vi "binning.vi"(10 "Number to bin":i32=2, 11 "path":path) -> ()   [LabVIEW 2023]
uses:
  <vilib>/Utility/file.llb/Read Delimited Spreadsheet (I64).vi
  <vilib>/Utility/file.llb/Write Delimited Spreadsheet (I64).vi
panel:
  out "Horizontal Fill Slide":dbl(slide) scale=0.0..100.0
  out "error out":errorcluster
  in  "error in":errorcluster
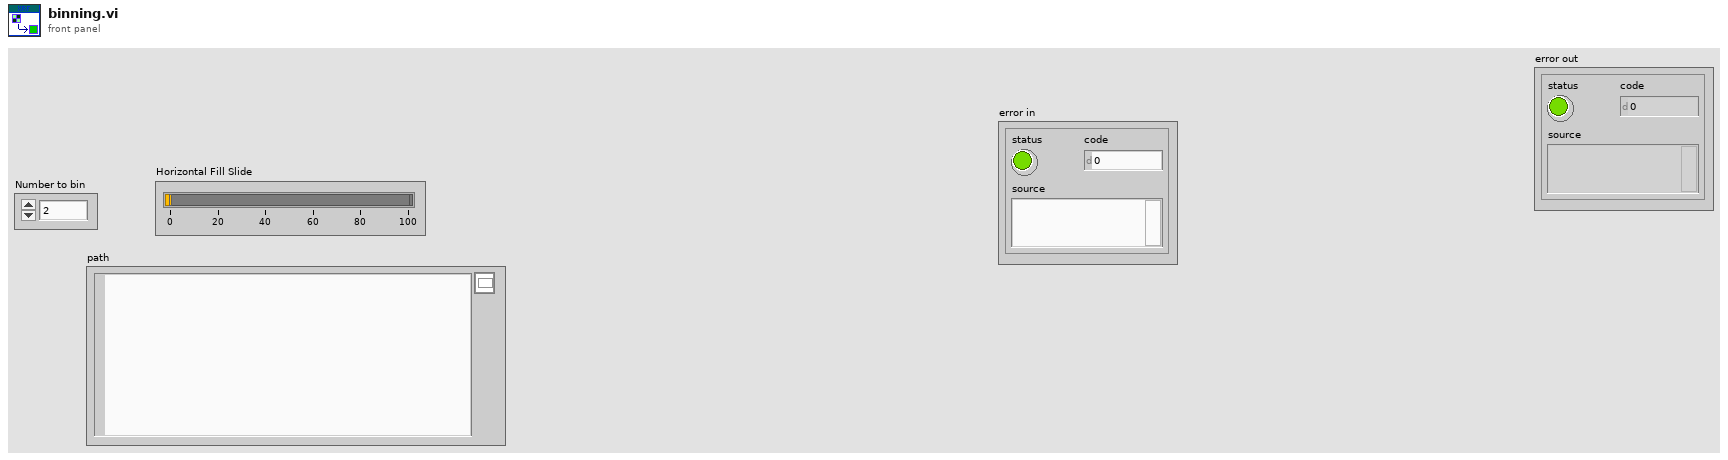
[diagram p1: front panel]
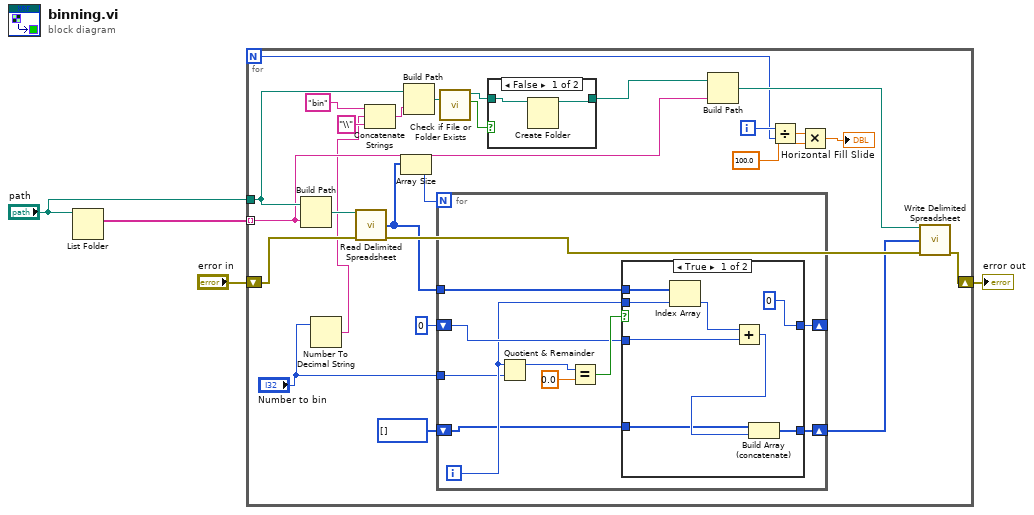
[diagram p0: block diagram]
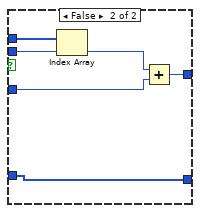
[diagram p3: hidden frame]
diagram:
  n1 = List Folder(path="path") -> (filenames=w4:string[])  [unwired: 3 in, 3 out]
  n2 = for {
    N -> [w20]
    tunnel: w4 -> [w12] mode=indexing
    tunnel: "path" -> [w13]
    shift-right: [w26] -> w1
    shift-left: "error in" -> [w28]
    i -> [w21]
    n3 = Build Path(base path=w13, name or relative path=w12) -> (appended path=w30:path)
    n4 = Number To Decimal String(number="Number to bin") -> (decimal integer string=w5:string)  [unwired: 1 in]
    n5 = call-poly <vilib>:"Read Delimited Spreadsheet.vi"("file path (dialog if empty)"=w30, "error in (no error)"=w28) -> ("first row"=w25:i64[], "error out"=w27:errorcluster)  [unwired: 8 in, 4 out]
    n6 = Concatenate Strings("bin" ("string"), w5, "\\" ("string")) -> (w9:string)
    n7 = Array Size(array=w25) -> (size(s)=w24:i32)
    n8 = Build Path(base path=w13, name or relative path=w9) -> (appended path=w16:path)
    n9 = for {
      N: w24 -> [_]
      tunnel: w25 -> [w43]
      shift-right: [w36] -> w22
      shift-left: i64[] [] -> [w35]
      shift-right: [w42] -> _
      shift-left: i64 0 ("Numeric") -> [w38]
      tunnel: "Number to bin" -> [w34]
      i -> [w37]
      n10 = Quotient & Remainder(x=w37, y=w34) -> (x-y*floor(x/y)=w41:i32)  [unwired: 1 out]
      n11 = Equal?(x=w41, y=0.0) -> (x = y?=w39:bool)
      n12 = case shown="True" w39 {
        tunnel: w43 -> [w51 w55]
        tunnel: [i64 0 ("Numeric") w54] -> w42
        tunnel: w37 -> [w50 w57]
        tunnel: w38 -> [w48 w52]
        tunnel: [w46 w56] -> w36
        tunnel: w35 -> [w44 w56]
        frame True {
          n13 = Index Array(array=w51, index=w50) -> (element=w49:i64)
          n14 = Add(x=w49, y=w48) -> (x+y=w45:i64)
          n15 = Build Array (concatenate)(w44, w45) -> (w46:i64[])
        }
        frame False {
          n16 = Index Array(array=w55, index=w57) -> (element=w53:i64)
          n17 = Add(x=w53, y=w52) -> (x+y=w54:i64)
        }
      }
    }
    n18 = call <vilib>:"Check if File or Folder Exists.vi"("path"=w16) -> ("file or folder exists?"=w14:bool, "dup path"=w15:path)  [unwired: 8 in, 1 out]
    n19 = case shown="False" w14 {
      tunnel: w15 -> [w32 w33]
      tunnel: [w31 w33] -> w11
      frame False {
        n20 = Create Folder(path (use dialog)=w32) -> (created path=w31:path)  [unwired: 2 in, 2 out]
      }
      frame True {
      }
    }
    n21 = Build Path(base path=w11, name or relative path=w12) -> (appended path=w29:path)
    n22 = Divide(x=w21, y=w20) -> (x/y=w19:dbl)
    n23 = Multiply(x=w19, y=100.0) -> (x*y=→"Horizontal Fill Slide":dbl)
    n24 = call-poly <vilib>:"Write Delimited Spreadsheet.vi"("file path (dialog if empty)"=w29, "1D data"=w22, "error in (no error)"=w27) -> ("error out"=w26:errorcluster)  [unwired: 11 in, 1 out]
  }
  "error out" <- w1
